vi "Save Notebook Before Opening One.vi"(11 "Not saved?":bool) -> (0 "Save?":bool, 3 "Save/Don't Save/Cancel":T1=enum."Button 2")   [LabVIEW 2021, in "Notebook.lvlib"]
uses:
  Notebook.lvlib
  GUI/3-Button Dialog Output.ctl
  GUI/GUI.lvlib
  Fits/Fits.lvlib
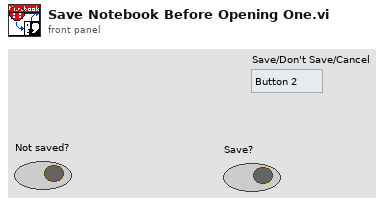
[diagram p1: front panel]
types:
  T1 = typedef "Fits.lvlib/3-Button Dialog Output.ctl" = enum16{"Window Close", "Button 1", "Button 2", "Button 3"}
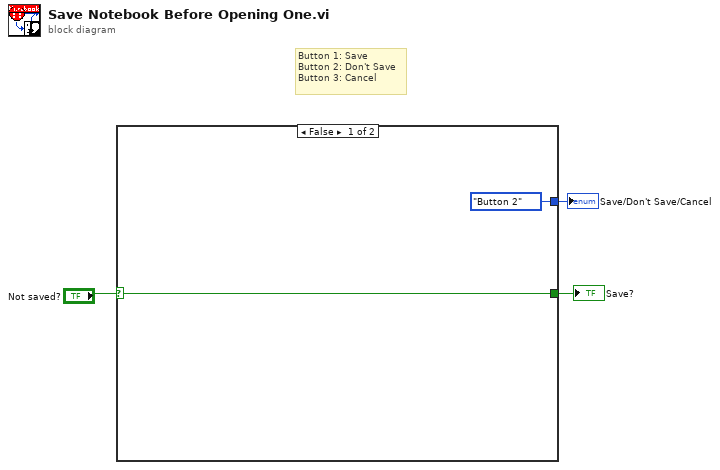
[diagram p0: block diagram]
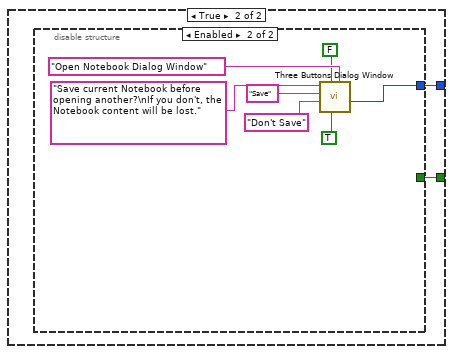
[diagram p2: hidden frame]
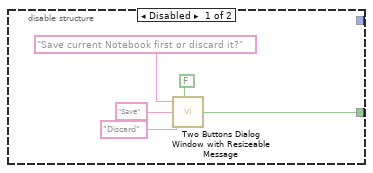
[diagram p3: hidden frame]
diagram:
  # "Button 1: Save\nButton 2: Don't Save\nButton 3: Cancel"
  n1 = case shown="False" "Not saved?" {
    selector: "Not saved?" -> [w5 _]
    tunnel: [w5 w7] -> w2
    tunnel: [3-Button_Dialog_Output."Button 2" ("3-button Dialog Output") w6] -> w1
    frame False {
    }
    frame True {
      n2 = disable-structure shown="Enabled" {
        disable-tunnel: [w11 _] -> w7
        disable-tunnel: [_ w15] -> w6
        frame Disabled {
          n3 = call "Two Buttons Dialog Window with Resizeable Message.vi"("Message"="Save current Notebook first or discard it?" ("message"), "Return =  OK (T)"=FALSE, "OK Button Text"="Save" ("F button name (\"Cancel\")"), "Cancel Button Text"="Discard") -> ("OK?"=w11:bool)  [unwired: 5 in]
        }
        frame Enabled {
          n4 = call "Three Buttons Dialog Window.vi"("Window Title"="Open Notebook Dialog Window" ("Window Title (\"\")"), "ESC =  Button 3 (T)"=TRUE, "Return =  Button 1 (T)"=FALSE, "Button 2 Text"="Don't Save" ("Center Button Text (\"No\")"), "Button 1 Text (OK)"="Save" ("Left Button Text (\"Yes\")"), "Message"="Save current Notebook before opening another?\nIf you don't, the Notebook content will be lost." ("message")) -> ("3-button Dialog Output"=w15:T1)  [unwired: 5 in]
        }
      }
    }
  }
  "Save?" <- w2
  "Save/Don't Save/Cancel" <- w1
